vi "DAQmx产生脉冲.vi"() -> ()   [LabVIEW 2010]
panel:
  in  "stop":bool
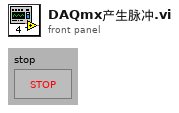
[diagram p1: front panel]
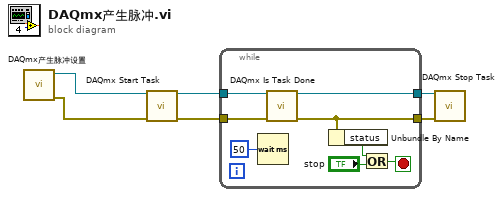
[diagram p0: block diagram]
diagram:
  n1 = call "DAQmx产生脉冲设置.vi"() -> ("error out"=w1:errorcluster, "task out"=w2:refnum<k21>)  [unwired: 10 in]
  n2 = call <vilib>:"DAQmx Start Task.vi"("task/channels in"=w2, "error in"=w1) -> ("task out"=w5:refnum<k21>, "error out"=w6:errorcluster)  [unwired: 12 in]
  n3 = while "Check for errors or stop pressed" {
    tunnel: w6 -> [w10]
    tunnel: [w11] -> w4
    tunnel: w5 -> [w12]
    tunnel: [w8] -> w3
    stop <- w13 stop-if-true
    n4 = Wait (ms)(milliseconds to wait=u32 50) -> ()  [unwired: 1 out]
    n5 = call <vilib>:"DAQmx Is Task Done.vi"("task/channels in"=w12, "error in"=w10) -> ("task out"=w11:refnum<k21>, "error out"=w8:errorcluster)  [unwired: 11 in, 1 out]
    n6 = Unbundle By Name(w8) -> ("status"=w9:bool)
    n7 = Or(x=w9, y="stop") -> (x .or. y?=w13:bool)
  }
  n8 = call <vilib>:"DAQmx Stop Task.vi"("task/channels in"=w4, "error in"=w3) -> ()  [unwired: 12 in, 2 out]
